vi "niDTS WLAN Dut Data Reset Inits.vi"(8 "error in (no error)":errorcluster, 11 "niDTS WLAN Dut Data in":refnum<class "niDTS WLAN Dut Data.lvclass">) -> (0 "error out":errorcluster, 3 "niDTS WLAN Dut Data out":refnum<class "niDTS WLAN Dut Data.lvclass">)   [LabVIEW 2015, in "niDTS WLAN.lvlib" / "niDTS WLAN Dut Data.lvclass"]
uses:
  niDTS WLAN Dut Data.lvclass
  niDTS WLAN Dut Data.lvclass/niDTS WLAN Dut Data.ctl
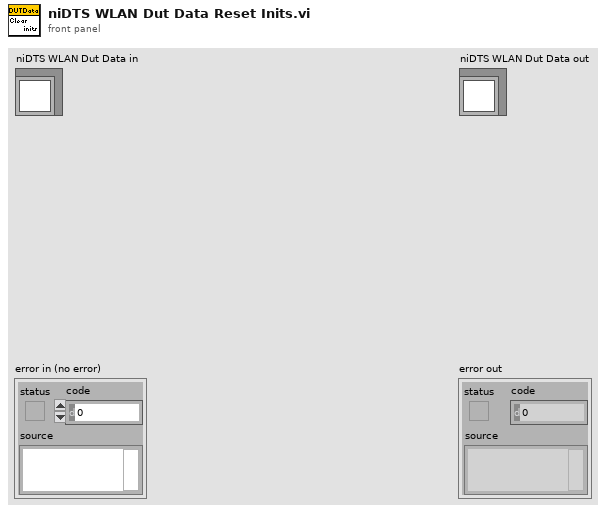
[diagram p1: front panel]
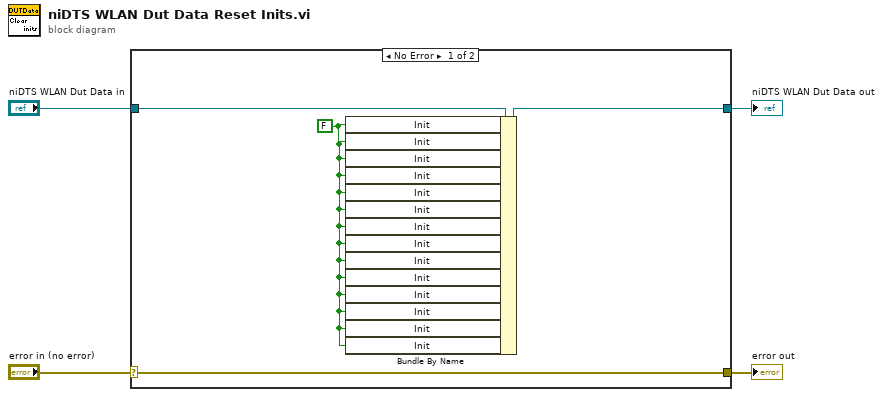
[diagram p0: block diagram]
diagram:
  n1 = case shown="No Error" "error in (no error)" {
    selector: "error in (no error)" -> [w7 w10]
    tunnel: [w7 w10] -> w3
    tunnel: [w6 w9] -> w1
    tunnel: "niDTS WLAN Dut Data in" -> [w8 w9]
    frame No Error {
      w5 = FALSE ("WLAN Type.Init")
      n2 = Bundle By Name(cluster=w8, "Init"=w5, "Init"=w5, "Init"=w5, "Init"=w5, "Init"=w5, "Init"=w5, "Init"=w5, "Init"=w5, "Init"=w5, "Init"=w5, "Init"=w5, "Init"=w5, "Init"=w5, "Init"=w5) -> (w6:refnum<class "niDTS WLAN Dut Data.lvclass">)
    }
    frame Error {
    }
  }
  "error out" <- w3
  "niDTS WLAN Dut Data out" <- w1
